vi "Test_PowerShell.vi"   [LabVIEW 2016]
uses:
  <vilib>/addons/_JKI Toolkits/Caraya/classes/Test/Test.lvclass
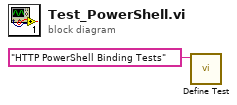
[diagram p0: block diagram]
diagram:
  n1 = call <vilib>:"Define Test.vi"("Label (VI Title)"="HTTP PowerShell Binding Tests") -> ()  [unwired: 10 in, 1 out]
